vi "Predicting Cost.vi"() -> ()   [LabVIEW 2023]
doc: "Determines the estimated total cost (in US dollars) of scone production based on the quantity of scones (X1) and the price of one pound of flour (X2). The General Linear Fit VI determines the coefficients used in the cost-estimate equation:\n\nY = b0 + b1X1 + b2X2\n\nTo use the General Linear Fit VI, the only parameters that you need to build are H (observation matrix) and Y Values. Each column of H is the observed data for each independent variable: the first column is 1 because the coefficient b0 is not associated with any independent variable. \n\nThe observed data would normally appear in three arrays (Y, X1, and X2). The block diagram shows how to build H for input to the General Linear Fit VI.\n\nThe resulting equation for the total cost of scone production becomes Y = -20.34 + 0.38X1 + 19.05X2."
uses:
  <vilib>/Analysis/NI_AALPro.lvlib
panel:
  out "Waveform Graph":dbl[][](graph)
  out "H":dbl[][](array[numeric])
  out "Equation":string
  out "mse":dbl
  out "Coefficients":dbl[](array[numeric])
  in  "X2":dbl[](array[numeric])=[3.0, 3.2, 3.1, 2.8, 2.5]
  in  "X1":dbl[](array[numeric])=[295.0, 100.0, 200.0, 700.0, 60.0]
  in  "Y":dbl[](array[numeric])=[150.0, 75.0, 120.0, 300.0, 50.0]
  # "Overview: Demonstrates the use of the General Linear Fit VI to predict cost.\nRequirements: LabVIEW Full Development System\nInstructions: \n1. Run the VI. \n2. Observe the fit equation and the H matrix structure.\n3. Open the block diagram and observe the construction of the H matrix."
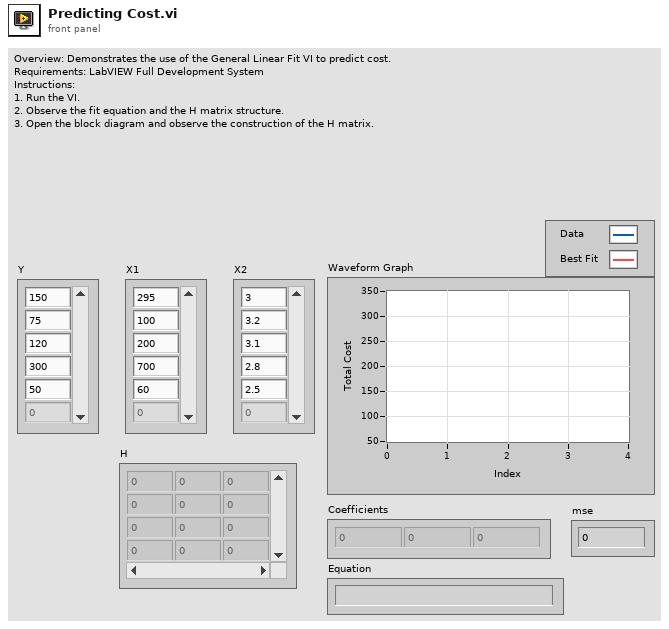
[diagram p1: front panel]
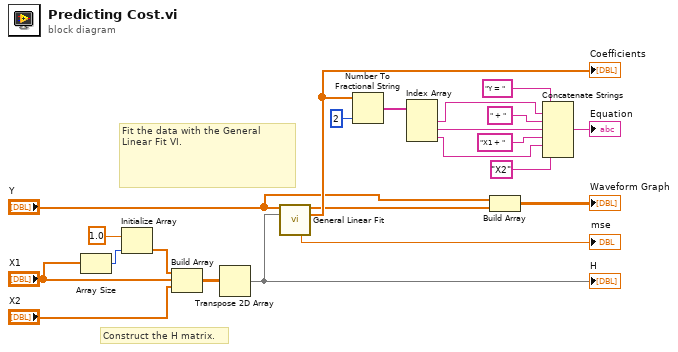
[diagram p0: block diagram]
diagram:
  # "Construct the H matrix."
  # "Fit the data with the General Linear Fit VI."
  n1 = Array Size(array="X1") -> (size(s)=w22:i32)
  n2 = Initialize Array(1.0, w22) -> (w20:dbl[])
  n3 = Build Array(w20, "X1", "X2") -> (w17:dbl[][])
  n4 = Transpose 2D Array(2D array=w17) -> (transposed array=w21:dbl[][])
  "H" <- w21
  n5 = call <vilib>:"General Linear Fit.vi"("Y"="Y", "H"=w21) -> ("Best Fit"=w4:dbl[], "Coefficients"=w10:dbl[], "residue"=→"mse":dbl)  [unwired: 8 in, 3 out]
  "Coefficients" <- w10
  n6 = Number To Fractional String(number=w10, precision (6)=2) -> (F-format string=w9:string[])  [unwired: 2 in]
  n7 = Index Array(array=w9) -> (element #1=w8:string, element #2=w7:string, element #3=w6:string)  [unwired: 3 in]
  n8 = Build Array("Y", w4) -> (→"Waveform Graph":dbl[][])
  n9 = Concatenate Strings("Y = ", w8, " + ", w7, "X1 + ", w6, "X2") -> (→"Equation":string)
